vi "Assign LS Timing.vi"(8 "error in (no error)":errorcluster, 10 "MasterTimingInfo":T1, 11 "Chassis Tasks in":refnum<class "Chassis Tasks.lvclass">) -> (0 "error out":errorcluster, 3 "Chassis Tasks out":refnum<class "Chassis Tasks.lvclass">)   [LabVIEW 2012]
uses:
  Chassis Tasks.lvclass
  SubVIs Main/SubVIs DAQ/Custom Ctrls/ge_MasterTimingInfo.ctl
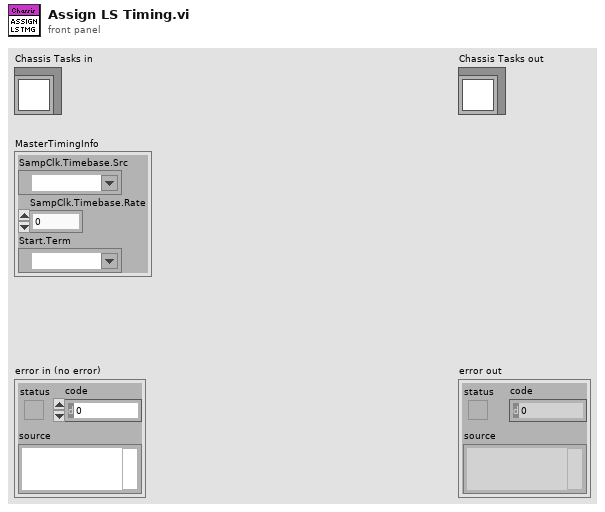
[diagram p1: front panel]
types:
  T1 = typedef "ge_MasterTimingInfo.ctl" = cluster{"SampClk.Timebase.Src":tag, "SampClk.Timebase.Rate":dbl, "Start.Term":tag}
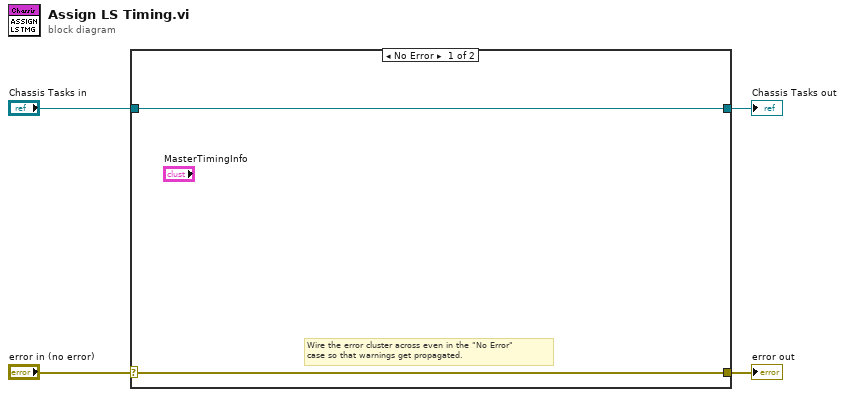
[diagram p0: block diagram]
diagram:
  n1 = case shown="No Error" "error in (no error)" {
    selector: "error in (no error)" -> [w5 w8]
    tunnel: [w5 w8] -> w3
    tunnel: [w6 w7] -> w1
    tunnel: "Chassis Tasks in" -> [w6 w7]
    frame No Error {
      # "Wire the error cluster across even in the \"No Error\"\ncase so that warnings get propagated."
    }
    frame Error {
    }
  }
  "error out" <- w3
  "Chassis Tasks out" <- w1
